vi "prueba_DB.vi"() -> ()   [LabVIEW 2014]
uses:
  <vilib>/addons/database/Auxilliary.llb/DB Tools Transaction.ctl
  <vilib>/addons/database/Auxilliary.llb/DB Tools Column Info.ctl
  <vilib>/addons/database/Auxilliary.llb/DB Tools DataTypes.ctl
  <vilib>/addons/database/Connection.llb/DB Tools Open Connec (String).vi
  <vilib>/addons/database/Connection.llb/Conn Transaction.vi
  <vilib>/addons/database/Auxilliary.llb/DB Tools Format Datetime String (Time Stamp).vi
  <vilib>/addons/database/_DB Variant To Data/Database Variant To Data.xnode
  <vilib>/addons/database/NI_Database_API.lvlib
panel:
  in  "Create Table?":bool
  out "error out":errorcluster
  in  "error in (no error)":errorcluster
  out "Tiempo en Seg.":dbl
  in  "table":string="win1"
  in  "prompt? (F)":bool
  in  "Delete Table?":bool
  out "tables":string[](array[string])
  out "Table Control":string[][](table)
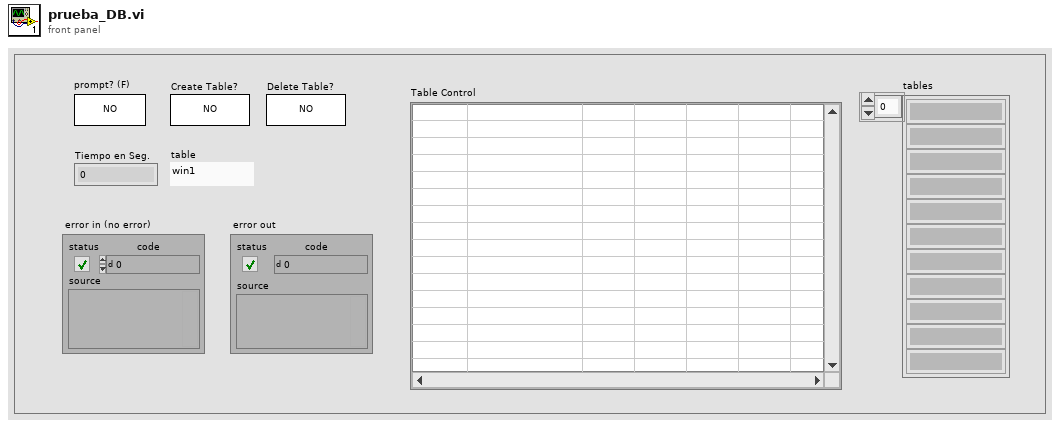
[diagram p1: front panel]
types:
  T1 = typedef "NI_Database_API.lvlib/DB Tools Transaction.ctl" = enum16{"begin", "commit", "rollback"}
  T2 = typedef "NI_Database_API.lvlib/DB Tools Column Info.ctl" = cluster{"column name":string, "data type":T3, "size":i32, "allow null?":bool}
  T3 = typedef "NI_Database_API.lvlib/DB Tools DataTypes.ctl" = enum16{"String", "Long (I32)", "Single (SGL)", "Double (DBL)", "Date/Time", "Binary"}
  T4 = typedef "NI_Database_API.lvlib/Conn ObjectReference.ctl" = refnum<k1>
  T5 = cluster{i32, "date/time string":string, bool, dbl}
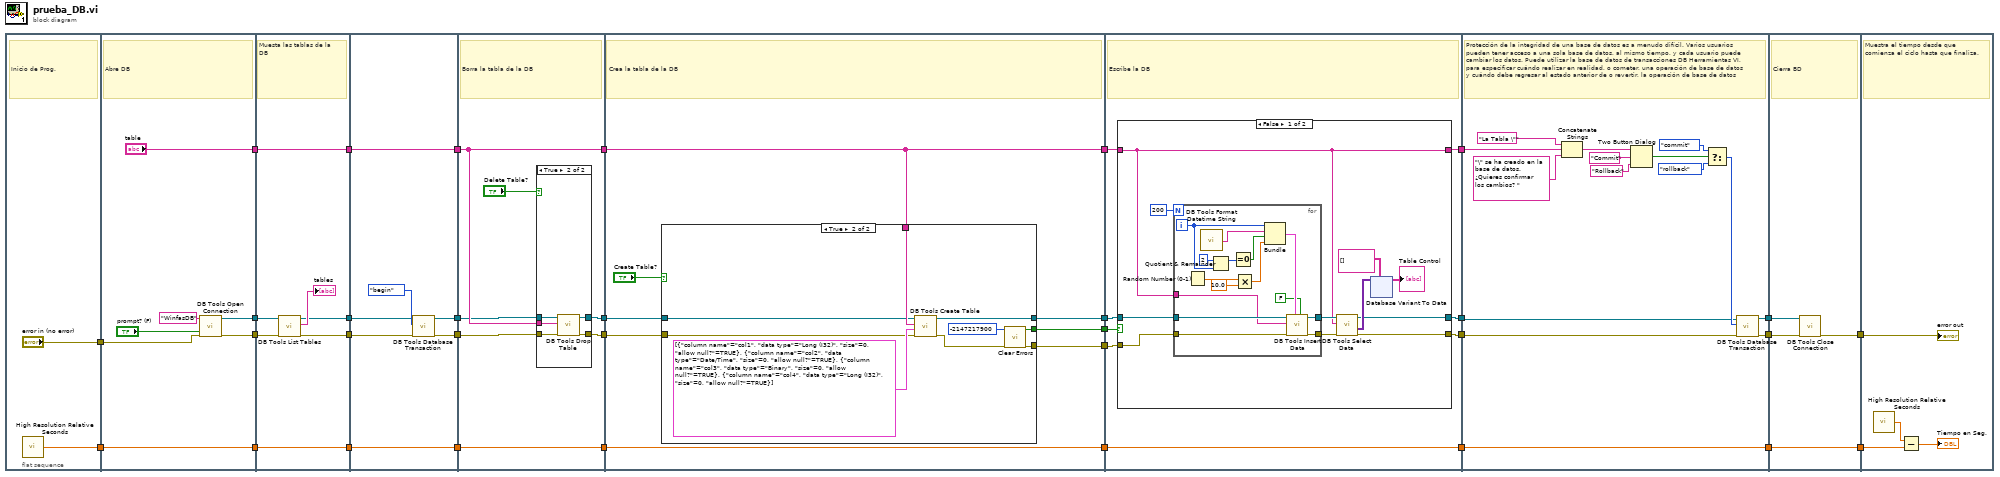
[diagram p0: block diagram]
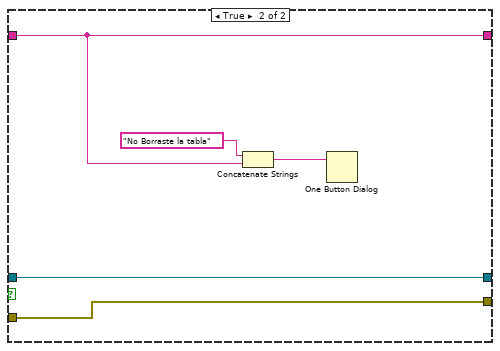
[diagram p4: hidden frame]
diagram:
  n1 = flat-sequence {
    tunnel: [w34] -> w32
    tunnel: ["error in (no error)"] -> w31
    tunnel: w32 -> [w39]
    tunnel: [w39] -> w9
    tunnel: w31 -> [w38]
    tunnel: ["table"] -> w7
    tunnel: [w36] -> w5
    tunnel: [w35] -> w4
    tunnel: w9 -> [w48]
    tunnel: [w48] -> w8
    tunnel: w7 -> [w47]
    tunnel: [w47] -> w6
    tunnel: w5 -> [w45]
    tunnel: w4 -> [w44]
    tunnel: [w43] -> w3
    tunnel: [w42] -> w2
    tunnel: w8 -> [w55]
    tunnel: [w55] -> w13
    tunnel: w6 -> [w54]
    tunnel: [w54] -> w12
    tunnel: [w50] -> w11
    tunnel: [w51] -> w10
    tunnel: w3 -> [w49]
    tunnel: w2 -> [w52]
    tunnel: w13 -> [w62]
    tunnel: [w62] -> w17
    tunnel: [w60] -> w16
    tunnel: [w61] -> w15
    tunnel: w12 -> [w59]
    tunnel: [w59] -> w14
    tunnel: w11 -> [w56]
    tunnel: w10 -> [w57]
    tunnel: w17 -> [w77]
    tunnel: [w77] -> w22
    tunnel: w16 -> [w76]
    tunnel: w15 -> [w73]
    tunnel: [w72] -> w21
    tunnel: w14 -> [w74]
    tunnel: [w74] -> w20
    tunnel: [w75] -> w19
    tunnel: [w70] -> w1
    tunnel: w22 -> [w96]
    tunnel: [w96] -> w28
    tunnel: [w94] -> w26
    tunnel: [w95] -> w24
    tunnel: w21 -> [w92]
    tunnel: w20 -> [w91]
    tunnel: w19 -> [w93]
    tunnel: [w90] -> w18
    tunnel: w1 -> [w89]
    tunnel: w28 -> [w186]
    tunnel: [w186] -> w27
    tunnel: w26 -> [w173]
    tunnel: [w184] -> w25
    tunnel: w24 -> [w174]
    tunnel: [w185] -> w23
    tunnel: w18 -> [w172]
    tunnel: w27 -> [w190]
    tunnel: [w190] -> w30
    tunnel: w25 -> [w188]
    tunnel: [w187] -> w29
    tunnel: w23 -> [w189]
    tunnel: w30 -> [w193]
    tunnel: w29 -> [w191]
    frame #0 {
      # "Inicio de Prog."
      n2 = call <vilib>:"High Resolution Relative Seconds.vi"() -> ("relative seconds"=w34:dbl)
    }
    frame #1 {
      # "Abre DB"
      n3 = call-poly <vilib>:"DB Tools Open Connection.vi"("error in (no error)"=w38, "prompt? (F)"="prompt? (F)", "connection information"="WinfasDB") -> ("error out"=w35:errorcluster, "connection reference"=w36:T4)  [unwired: 5 in]
    }
    frame #2 {
      # "Muesta las tablas de la DB"
      n4 = call <vilib>:"DB Tools List Tables.vi"("error in (no error)"=w44, "connection reference"=w45) -> ("error out"=w43:errorcluster, "tables"=→"tables":string[], "connection reference out"=w42:T4)  [unwired: 3 in]
    }
    frame #3 {
      n5 = call-poly <vilib>:"DB Tools Database Transaction.vi"("error in (no error)"=w49, "operation (begin)"=DB_Tools_Transaction."begin", "connection reference"=w52) -> ("error out"=w51:errorcluster, "connection reference out"=w50:T4)  [unwired: 3 in]
    }
    frame #4 {
      # "Borra la tabla de la DB"
      n6 = case shown="True" "Delete Table?" {
        tunnel: [w63 w69] -> w60
        tunnel: [w64 w68] -> w61
        tunnel: w57 -> [w63 w67]
        tunnel: w56 -> [w64 w66]
        tunnel: w59 -> [_ w65]
        frame False {
        }
        frame True {
          n7 = call <vilib>:"DB Tools Drop Table.vi"("error in (no error)"=w67, "table"=w65, "connection reference"=w66) -> ("error out"=w69:errorcluster, "connection reference out"=w68:T4)  [unwired: 5 in]
        }
      }
    }
    frame #5 {
      # "Crea la tabla de la DB"
      n8 = case shown="True" "Create Table?" {
        tunnel: w76 -> [w78 w85]
        tunnel: [w78 w84] -> w75
        tunnel: [_ w83] -> w70
        tunnel: w74 -> [_ w82]
        tunnel: w73 -> [w79 w81]
        tunnel: [w79 w80] -> w72
        frame False {
        }
        frame True {
          n9 = call <vilib>:"DB Tools Create Table.vi"("error in (no error)"=w85, "column information"=T2[] [{"column name"="col1", "data type"=enum."Long (I32)", "size"=0, "allow null?"=TRUE}, {"column name"="col2", "data type"=enum."Date/Time", "size"=0, "allow null?"=TRUE}, {"column name"="col3", "data type"=enum."Binary", "size"=0, "allow null?"=TRUE}, {"column name"="col4", "data type"=enum."Long (I32)", "size"=0, "allow null?"=TRUE}], "table"=w82, "connection reference"=w81) -> ("error out"=w87:errorcluster, "connection reference out"=w80:T4)  [unwired: 4 in]
          n10 = call <vilib>:"Clear Errors.vi"("error in (no error)"=w87, "specific error code to clear (0: all)"=-2147217900) -> ("error out"=w84:errorcluster, "specific error cleared?"=w83:bool)  [unwired: 4 in]
        }
      }
    }
    frame #6 {
      # "Escribe la DB"
      n11 = case shown="False" w89 {
        tunnel: w92 -> [w107 w171]
        tunnel: w91 -> [w97 w167]
        tunnel: w93 -> [w102 w170]
        tunnel: [w100 w170] -> w94
        tunnel: [w101 w171] -> w95
        tunnel: [w97 w167] -> w90
        frame False {
          n12 = for {
            N: 200 -> [_]
            tunnel: w107 -> [w165]
            tunnel: [w164] -> w99
            tunnel: w102 -> [w166]
            tunnel: [w163] -> w98
            tunnel: w97 -> [w157]
            i -> [w161]
            n13 = Random Number (0-1)() -> (number: 0 to 1=w155:dbl)
            n14 = call-poly <vilib>:"DB Tools Format Datetime String.vi"() -> ("date/time string"=w152:string)  [unwired: 1 in]
            n15 = Quotient & Remainder(x=2, y=w161) -> (x-y*floor(x/y)=w156:i32)  [unwired: 1 out]
            n16 = Equal To 0?(x=w156) -> (x = 0?=w159:bool)
            n17 = Multiply(x=w155, y=10.0) -> (x*y=w154:dbl)
            n18 = Bundle(w161, "date/time string"=w152, w159, w154) -> (w162:T5)  [unwired: 1 in]
            n19 = call <vilib>:"DB Tools Insert Data.vi"("create table? (F)"=FALSE, "data"=w162, "error in (no error)"=w166, "table"=w157, "connection reference"=w165) -> ("error out"=w163:errorcluster, "connection reference out"=w164:T4)  [unwired: 5 in]
          }
          n20 = call <vilib>:"DB Tools Select Data.vi"("error in (no error)"=w98, "table"=w97, "connection reference"=w99) -> ("error out"=w100:errorcluster, "data"=w105:variant[][], "connection reference out"=w101:T4)  [unwired: 3 in]
          n21 = xnode "Database Variant To Data"("database variant"=w105, "type"=string[][] [] ("Table Control 2")) -> ("data"=→"Table Control":string[][])  [unwired: 1 in, 1 out]
        }
        frame True {
          n22 = Concatenate Strings("No Borraste la tabla" ("message"), w167) -> (w168:string)
          n23 = One Button Dialog(message=w168) -> ()  [unwired: 1 in, 1 out]
        }
      }
    }
    frame #7 {
      # "Protección de la integridad de una base de datos es a menudo difícil. Varios usuarios pueden tener acceso a una sola base de datos, al mismo tiempo, y cada usuario puede cambiar los datos. Puede utilizar la base de datos de transacciones DB Herramientas VI, para especificar cuándo realizar en realidad, o cometer, una operación de base de datos y cuándo debe regresar al estado anterior de o revertir, la operación de base de datos"
      n24 = Concatenate Strings("La Tabla \"" ("string"), w172, "\" se ha creado en la base de datos. ¿Quieres confirmar los cambios? " ("string")) -> (w181:string)
      n25 = Two Button Dialog(message=w181, 1:"Rollback" ("F button name (\"Cancel\")"), 2:"Commit" ("T button name (\"OK\")")) -> (T button?=w180:bool)
      n26 = Select(t=DB_Tools_Transaction."commit" ("operation (begin)"), s=w180, f=DB_Tools_Transaction."rollback" ("operation (begin)")) -> (s? t:f=w175:T1)
      n27 = call-poly <vilib>:"DB Tools Database Transaction.vi"("error in (no error)"=w173, "operation (begin)"=w175, "connection reference"=w174) -> ("error out"=w184:errorcluster, "connection reference out"=w185:T4)  [unwired: 3 in]
    }
    frame #8 {
      # "Cierra BD"
      n28 = call <vilib>:"DB Tools Close Connection.vi"("error in (no error)"=w188, "connection reference"=w189) -> ("error out"=w187:errorcluster)  [unwired: 5 in]
    }
    frame #9 {
      # "Muestra el tiempo desde que comienza el ciclo hasta que finaliza."
      n29 = call <vilib>:"High Resolution Relative Seconds.vi"() -> ("relative seconds"=w194:dbl)
      n30 = Subtract(x=w194, y=w193) -> (x-y=→"Tiempo en Seg.":dbl)
      "error out" <- w191
    }
  }
